vi "CreateNumberingHeader.vi"(11 "データ数":i32) -> (3 "連番ヘッダ":string[](array[string]))   [LabVIEW 2014]
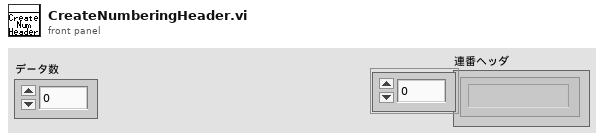
[diagram p1: front panel]
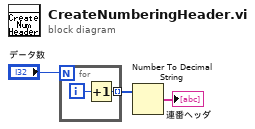
[diagram p0: block diagram]
diagram:
  n1 = for {
    N: "データ数" -> [_]
    tunnel: [w4] -> w2 mode=indexing
    i -> [w5]
    n2 = Increment(x=w5) -> (x+1=w4:i32)
  }
  n3 = Number To Decimal String(number=w2) -> (decimal integer string=→"連番ヘッダ":string[])  [unwired: 1 in]
